vi "UI Main Page.vi"(8 "error in":errorcluster) -> (0 "error out":errorcluster)   [LabVIEW 2019, in "UIs.lvlib"]
uses:
  UIs.lvlib
  <vilib>/Utility/miscctls.llb/LVPointTypeDef.ctl
  User Event/Controls/UE Abort Action.ctl
  Controller/Controller.lvlib
  Test/Test.lvlib
panel:
  in  "I/O":bool
  in  "Camera":bool
  in  "Laser":bool
  in  "Tubing Install":bool
  in  "Air Tight":bool
  in  "Chip Fitting":bool
  in  "Selection Valve":bool
  in  "Limit Sensor":bool
  in  "Flow Rate of Wash Tank":bool
  in  "Flow Rate of Buffer Tank":bool
  in  "Flow Field/Flow Rate":bool
  in  "Exit":bool
  # "Functional Test"
  # "Fluidic Test"
  # "Optical Test"
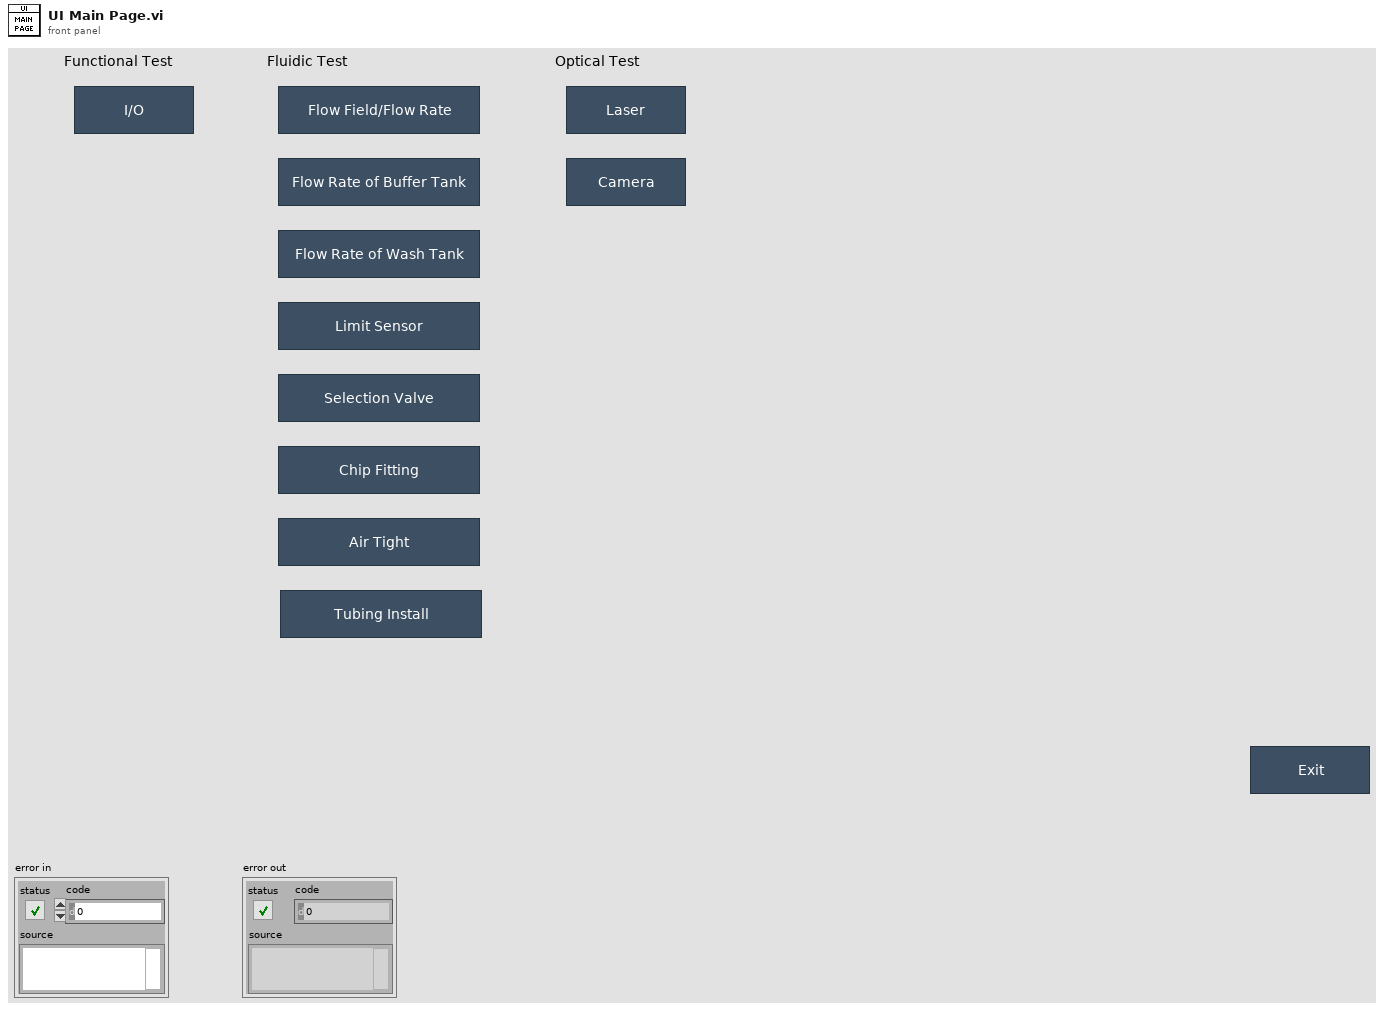
[diagram p1: front panel]
types:
  T1 = typedef "LVPointTypeDef.ctl" = cluster{"Horizontal":i16, "Vertical":i16}
  T2 = typedef "UE Abort Action.ctl" = enum16{"Create", "Get", "Destroy"}
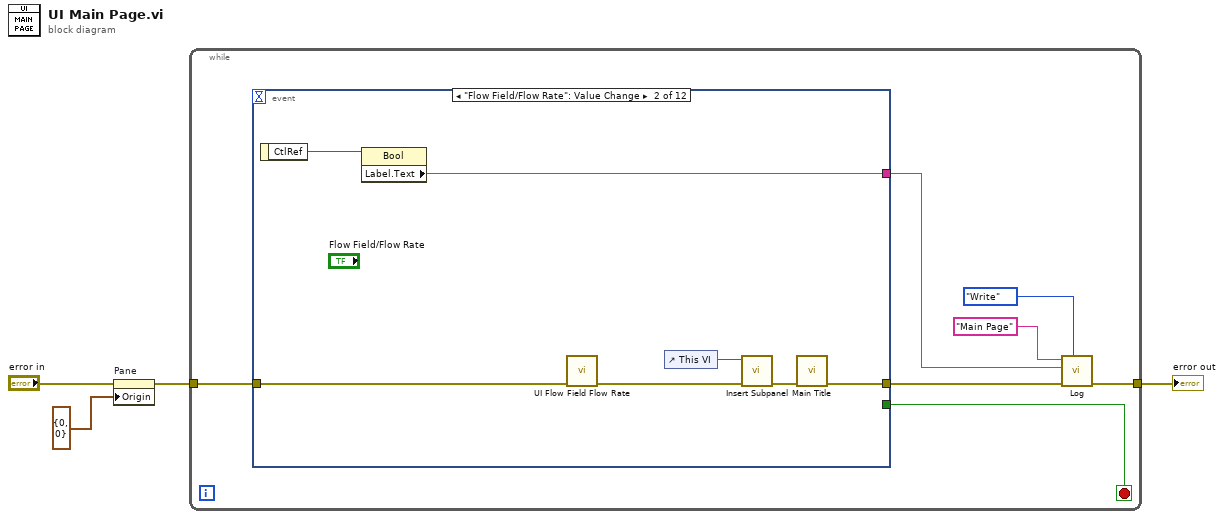
[diagram p0: block diagram]
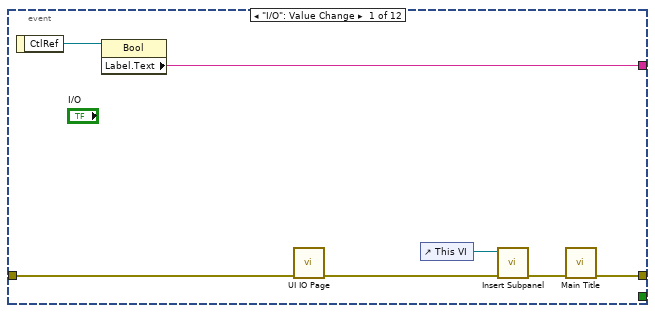
[diagram p2: hidden frame]
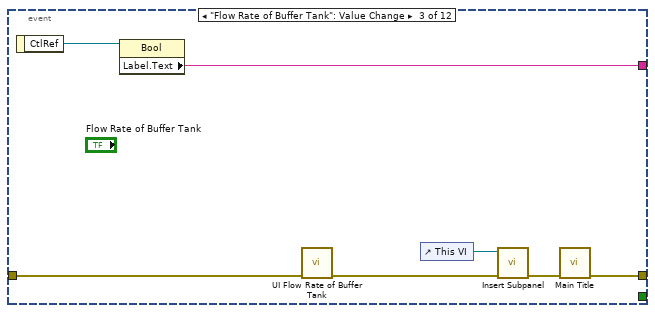
[diagram p3: hidden frame]
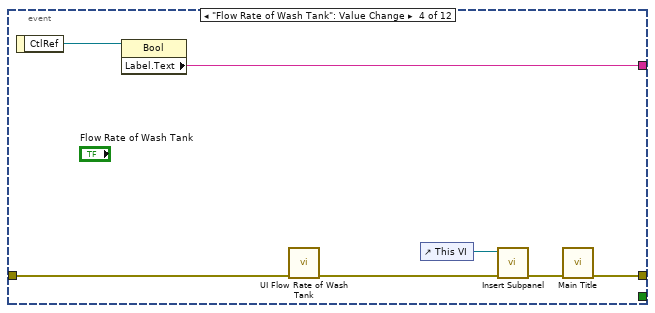
[diagram p4: hidden frame]
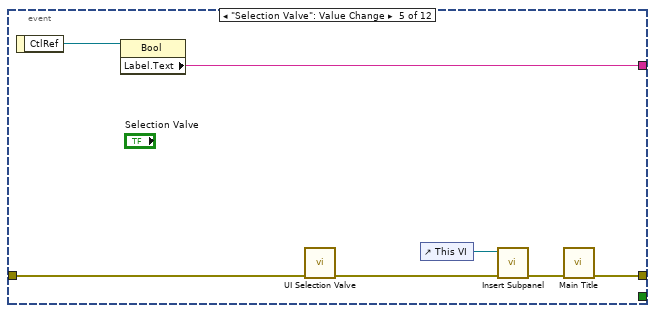
[diagram p5: hidden frame]
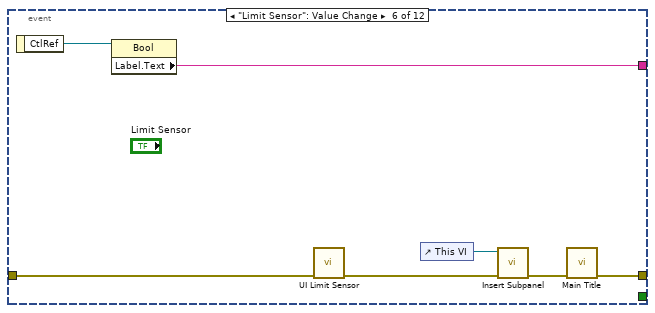
[diagram p6: hidden frame]
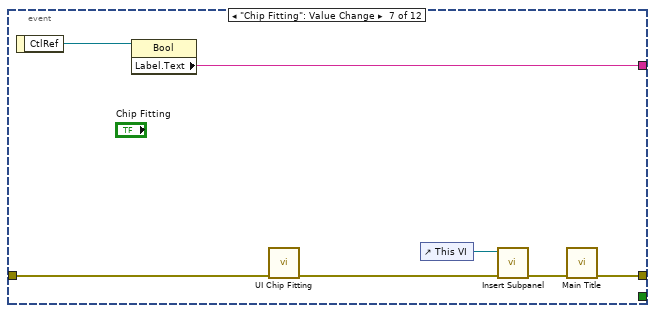
[diagram p7: hidden frame]
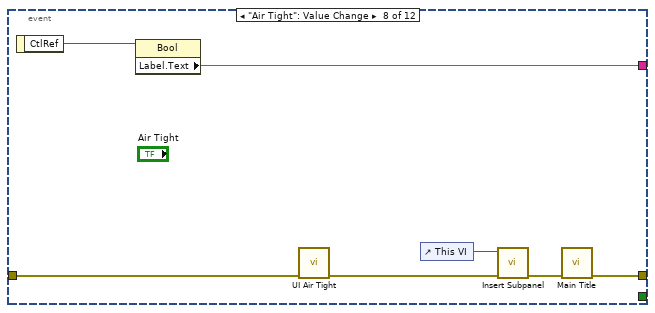
[diagram p8: hidden frame]
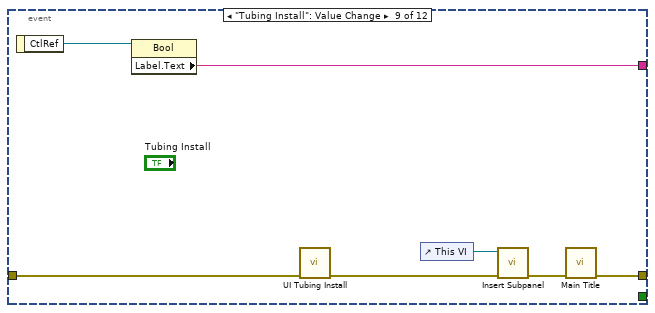
[diagram p9: hidden frame]
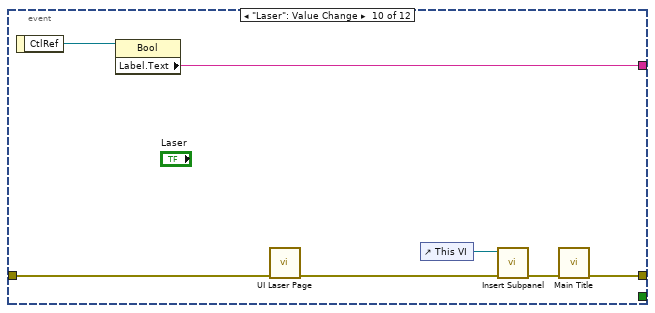
[diagram p10: hidden frame]
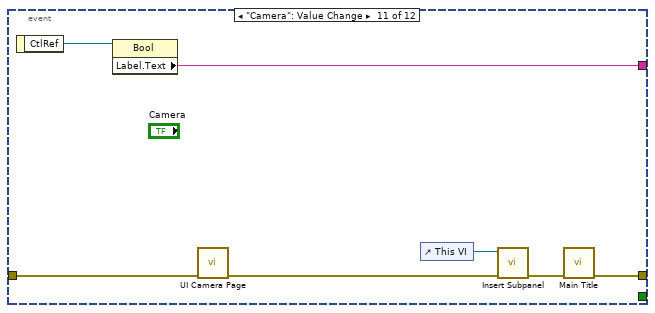
[diagram p11: hidden frame]
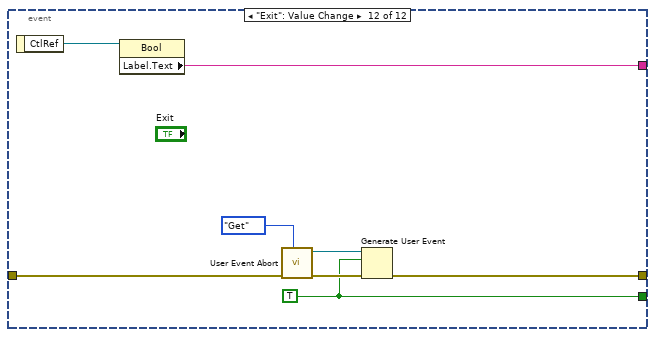
[diagram p12: hidden frame]
diagram:
  n1 = property on="Pane" class="Pane"(error in="error in", "Origin"=T1 {"Horizontal"=0, "Vertical"=0}) -> (error out=w2:errorcluster)  [unwired: 1 in, 1 out]
  n2 = while {
    tunnel: w2 -> [w11]
    tunnel: [w8] -> w4
    stop <- w10 stop-if-true
    n3 = event shown="[1] \"Flow Field/Flow Rate\": Value Change" {
      selector: _ -> [_ _ _ _ _ _ _ _ _ _ _ _]
      dyn-events: _ -> [_ _ _ _ _ _ _ _ _ _ _ _]
      timeout: _ -> [_ _ _ _ _ _ _ _ _ _ _ _]
      tunnel: w11 -> [w17 w24 w31 w38 w45 w52 w59 w66 w73 w80 w87 w93]
      tunnel: [_ _ _ _ _ _ _ _ _ _ _ w91] -> w10
      tunnel: [w14 w21 w28 w35 w42 w49 w56 w63 w70 w77 w84 w92] -> w9
      tunnel: [w12 w19 w26 w33 w40 w47 w54 w61 w68 w75 w82 w89] -> w6
      event "I/O": Value Change {
        n4 = event-data() -> ("CtlRef"=w13:refnum<vi>)  [unwired: 1 in]
        n5 = property class="Bool"(reference=w13) -> ("Label.Text"=w12:string)  [unwired: 1 in, 2 out]
        n6 = call "UI IO Page.vi"("error in"=w17) -> ("error out"=w16:errorcluster)  [unwired: 10 in]
        n7 = control-ref of="This VI"() -> (w18:refnum<vi>)
        n8 = call "Insert Subpanel.vi"("Error In"=w16, "VI Refnum"=w18) -> ("Error Out"=w15:errorcluster)  [unwired: 9 in]
        n9 = call "Main Title.vi"("Error In"=w15) -> ("Error Out"=w14:errorcluster)  [unwired: 10 in]
      }
      event "Flow Field/Flow Rate": Value Change {
        n10 = event-data() -> ("CtlRef"=w20:refnum<vi>)  [unwired: 1 in]
        n11 = property class="Bool"(reference=w20) -> ("Label.Text"=w19:string)  [unwired: 1 in, 2 out]
        n12 = call "UI Flow Field Flow Rate.vi"("error in"=w24) -> ("error out"=w23:errorcluster)  [unwired: 10 in]
        n13 = control-ref of="This VI"() -> (w25:refnum<vi>)
        n14 = call "Insert Subpanel.vi"("Error In"=w23, "VI Refnum"=w25) -> ("Error Out"=w22:errorcluster)  [unwired: 9 in]
        n15 = call "Main Title.vi"("Error In"=w22) -> ("Error Out"=w21:errorcluster)  [unwired: 10 in]
      }
      event "Flow Rate of Buffer Tank": Value Change {
        n16 = event-data() -> ("CtlRef"=w27:refnum<vi>)  [unwired: 1 in]
        n17 = property class="Bool"(reference=w27) -> ("Label.Text"=w26:string)  [unwired: 1 in, 2 out]
        n18 = call "UI Flow Rate of Buffer Tank.vi"("error in"=w31) -> ("error out"=w30:errorcluster)  [unwired: 10 in]
        n19 = control-ref of="This VI"() -> (w32:refnum<vi>)
        n20 = call "Insert Subpanel.vi"("Error In"=w30, "VI Refnum"=w32) -> ("Error Out"=w29:errorcluster)  [unwired: 9 in]
        n21 = call "Main Title.vi"("Error In"=w29) -> ("Error Out"=w28:errorcluster)  [unwired: 10 in]
      }
      event "Flow Rate of Wash Tank": Value Change {
        n22 = event-data() -> ("CtlRef"=w34:refnum<vi>)  [unwired: 1 in]
        n23 = property class="Bool"(reference=w34) -> ("Label.Text"=w33:string)  [unwired: 1 in, 2 out]
        n24 = call "UI Flow Rate of Wash Tank.vi"("error in"=w38) -> ("error out"=w37:errorcluster)  [unwired: 10 in]
        n25 = control-ref of="This VI"() -> (w39:refnum<vi>)
        n26 = call "Insert Subpanel.vi"("Error In"=w37, "VI Refnum"=w39) -> ("Error Out"=w36:errorcluster)  [unwired: 9 in]
        n27 = call "Main Title.vi"("Error In"=w36) -> ("Error Out"=w35:errorcluster)  [unwired: 10 in]
      }
      event "Selection Valve": Value Change {
        n28 = event-data() -> ("CtlRef"=w41:refnum<vi>)  [unwired: 1 in]
        n29 = property class="Bool"(reference=w41) -> ("Label.Text"=w40:string)  [unwired: 1 in, 2 out]
        n30 = call "UI Selection Valve.vi"("error in"=w45) -> ("error out"=w44:errorcluster)  [unwired: 10 in]
        n31 = control-ref of="This VI"() -> (w46:refnum<vi>)
        n32 = call "Insert Subpanel.vi"("Error In"=w44, "VI Refnum"=w46) -> ("Error Out"=w43:errorcluster)  [unwired: 9 in]
        n33 = call "Main Title.vi"("Error In"=w43) -> ("Error Out"=w42:errorcluster)  [unwired: 10 in]
      }
      event "Limit Sensor": Value Change {
        n34 = event-data() -> ("CtlRef"=w48:refnum<vi>)  [unwired: 1 in]
        n35 = property class="Bool"(reference=w48) -> ("Label.Text"=w47:string)  [unwired: 1 in, 2 out]
        n36 = call "UI Limit Sensor.vi"("error in"=w52) -> ("error out"=w51:errorcluster)  [unwired: 10 in]
        n37 = control-ref of="This VI"() -> (w53:refnum<vi>)
        n38 = call "Insert Subpanel.vi"("Error In"=w51, "VI Refnum"=w53) -> ("Error Out"=w50:errorcluster)  [unwired: 9 in]
        n39 = call "Main Title.vi"("Error In"=w50) -> ("Error Out"=w49:errorcluster)  [unwired: 10 in]
      }
      event "Chip Fitting": Value Change {
        n40 = event-data() -> ("CtlRef"=w55:refnum<vi>)  [unwired: 1 in]
        n41 = property class="Bool"(reference=w55) -> ("Label.Text"=w54:string)  [unwired: 1 in, 2 out]
        n42 = call "UI Chip Fitting.vi"("error in"=w59) -> ("error out"=w58:errorcluster)  [unwired: 10 in]
        n43 = control-ref of="This VI"() -> (w60:refnum<vi>)
        n44 = call "Insert Subpanel.vi"("Error In"=w58, "VI Refnum"=w60) -> ("Error Out"=w57:errorcluster)  [unwired: 9 in]
        n45 = call "Main Title.vi"("Error In"=w57) -> ("Error Out"=w56:errorcluster)  [unwired: 10 in]
      }
      event "Air Tight": Value Change {
        n46 = event-data() -> ("CtlRef"=w62:refnum<vi>)  [unwired: 1 in]
        n47 = property class="Bool"(reference=w62) -> ("Label.Text"=w61:string)  [unwired: 1 in, 2 out]
        n48 = call "UI Air Tight.vi"("error in"=w66) -> ("error out"=w65:errorcluster)  [unwired: 10 in]
        n49 = control-ref of="This VI"() -> (w67:refnum<vi>)
        n50 = call "Insert Subpanel.vi"("Error In"=w65, "VI Refnum"=w67) -> ("Error Out"=w64:errorcluster)  [unwired: 9 in]
        n51 = call "Main Title.vi"("Error In"=w64) -> ("Error Out"=w63:errorcluster)  [unwired: 10 in]
      }
      event "Tubing Install": Value Change {
        n52 = event-data() -> ("CtlRef"=w69:refnum<vi>)  [unwired: 1 in]
        n53 = property class="Bool"(reference=w69) -> ("Label.Text"=w68:string)  [unwired: 1 in, 2 out]
        n54 = call "UI Tubing Install.vi"("error in"=w73) -> ("error out"=w72:errorcluster)  [unwired: 10 in]
        n55 = control-ref of="This VI"() -> (w74:refnum<vi>)
        n56 = call "Insert Subpanel.vi"("Error In"=w72, "VI Refnum"=w74) -> ("Error Out"=w71:errorcluster)  [unwired: 9 in]
        n57 = call "Main Title.vi"("Error In"=w71) -> ("Error Out"=w70:errorcluster)  [unwired: 10 in]
      }
      event "Laser": Value Change {
        n58 = event-data() -> ("CtlRef"=w76:refnum<vi>)  [unwired: 1 in]
        n59 = property class="Bool"(reference=w76) -> ("Label.Text"=w75:string)  [unwired: 1 in, 2 out]
        n60 = call "UI Laser Page.vi"("error in"=w80) -> ("error out"=w79:errorcluster)  [unwired: 10 in]
        n61 = control-ref of="This VI"() -> (w81:refnum<vi>)
        n62 = call "Insert Subpanel.vi"("Error In"=w79, "VI Refnum"=w81) -> ("Error Out"=w78:errorcluster)  [unwired: 9 in]
        n63 = call "Main Title.vi"("Error In"=w78) -> ("Error Out"=w77:errorcluster)  [unwired: 10 in]
      }
      event "Camera": Value Change {
        n64 = event-data() -> ("CtlRef"=w83:refnum<vi>)  [unwired: 1 in]
        n65 = property class="Bool"(reference=w83) -> ("Label.Text"=w82:string)  [unwired: 1 in, 2 out]
        n66 = call "UI Camera Page.vi"("error in"=w87) -> ("error out"=w86:errorcluster)  [unwired: 10 in]
        n67 = control-ref of="This VI"() -> (w88:refnum<vi>)
        n68 = call "Insert Subpanel.vi"("Error In"=w86, "VI Refnum"=w88) -> ("Error Out"=w85:errorcluster)  [unwired: 9 in]
        n69 = call "Main Title.vi"("Error In"=w85) -> ("Error Out"=w84:errorcluster)  [unwired: 10 in]
      }
      event "Exit": Value Change {
        w91 = TRUE
        n70 = event-data() -> ("CtlRef"=w90:refnum<vi>)  [unwired: 1 in]
        n71 = property class="Bool"(reference=w90) -> ("Label.Text"=w89:string)  [unwired: 1 in, 2 out]
        n72 = call "User Event Abort.vi"("Action"=UE_Abort_Action."Get", "Error In"=w93) -> ("Error Out"=w96:errorcluster, "User Event Out"=w95:refnum<user-event>)  [unwired: 8 in]
        n73 = Generate User Event(user event=w95, event data cluster=w91, error in=w96) -> (error out=w92:errorcluster)  [unwired: 1 in, 1 out]
      }
    }
    n74 = call "Log.vi"("Action"=enum16{"None", "Write"}."Write", "error in"=w9, "State"=w6, "Page Name"="Main Page") -> ("error out"=w8:errorcluster)  [unwired: 7 in]
  }
  "error out" <- w4
